vi "Export Data to Clipboard.vi"() -> ()   [LabVIEW 2010]
uses:
  <vilib>/Utility/file.llb/Read From Spreadsheet File (I64).vi
panel:
  out "Data Array":i64[][](array[numeric])
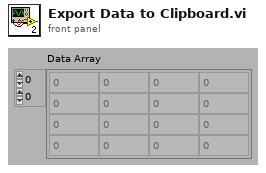
[diagram p1: front panel]
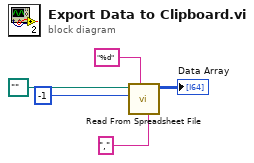
[diagram p0: block diagram]
diagram:
  n1 = call-poly <vilib>:"Read From Spreadsheet File.vi"("delimiter (\\t)"="," ("delimiter (\\t)"), "format (%d)"="%d", "number of rows (all:-1)"=-1, "file path (dialog if empty)"=path "" ("new file path (Not A Path if cancelled)")) -> ("all rows"=→"Data Array":i64[][])  [unwired: 3 in, 4 out]
